vi "Set CUR wrapper.vi"(7 "bAckEna":i32, 8 "error in (no error)":errorcluster caption="错误输入（无错误）", 9 "fCUR":dbl, 10 "dwCanNodeId":u32, 11 "dwDevIndex":u32) -> (0 "error out":errorcluster caption="错误输出", 3 "function return":u32, 4 "pACKInfo out":T1)   [LabVIEW 2016, in "UISimCanFunc_wrapper.lvlib"]
doc: "_declspec (dllexport) DWORD SetCUR_wrapper(DWORD dwDevIndex, DWORD dwCanNodeId, INT iCUR, BOOL bAckEna, P_BASIC_ACK_OBJ pACKInfo);"
uses:
  <userlib>/UISimCanFunc_wrapper/UISimCanFunc_wrapper.lvlib
  <userlib>/UISimCanFunc_wrapper/UISimCanFunc_wrapper.dll
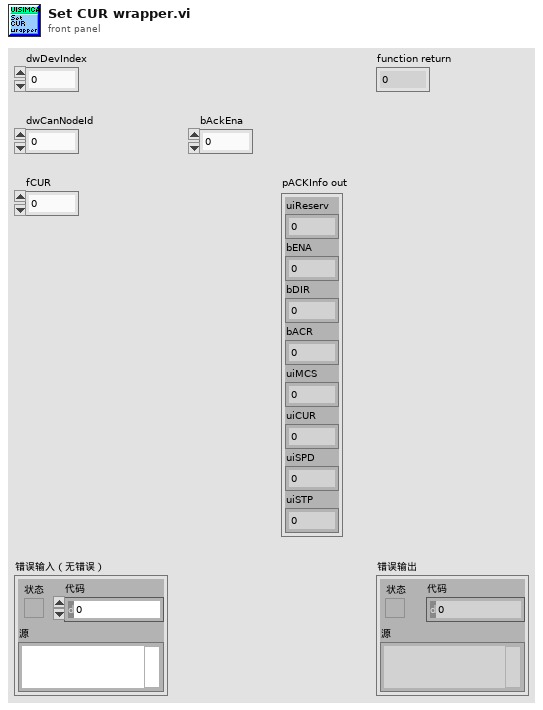
[diagram p1: front panel]
types:
  T1 = cluster{"uiReserv":u32, "bENA":i32, "bDIR":i32, "bACR":i32, "uiMCS":u32, "uiCUR":u32, "uiSPD":u32, "uiSTP":u32}
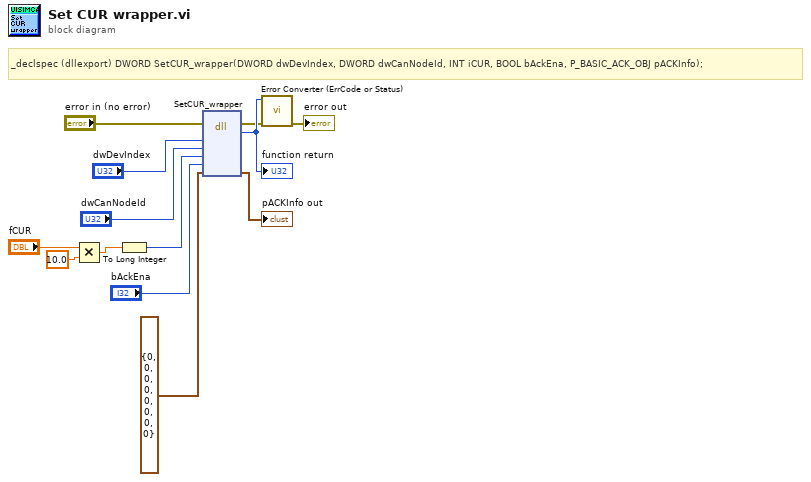
[diagram p0: block diagram]
diagram:
  # "_declspec (dllexport) DWORD SetCUR_wrapper(DWORD dwDevIndex, DWORD dwCanNodeId, INT iCUR, BOOL bAckEna, P_BASIC_ACK_OBJ pACKInfo);"
  n1 = Multiply(x="fCUR", y=10.0) -> (x*y=w2:dbl)
  n2 = To Long Integer(number=w2) -> (32bit integer=w1:i32)
  n3 = dll-call lib="C:/Program Files (x86)/National Instruments/LabVIEW 2016/user.lib/UISimCanFunc_wrapper/UISimCanFunc_wrapper.*" fn="SetCUR_wrapper"(error in="error in (no error)", "dwDevIndex"="dwDevIndex", "dwCanNodeId"="dwCanNodeId", "iCUR"=w1, "bAckEna"="bAckEna", "pACKInfo"=T1 {"uiReserv"=0, "bENA"=0, "bDIR"=0, "bACR"=0, "uiMCS"=0, "uiCUR"=0, "uiSPD"=0, "uiSTP"=0}) -> (error out=w6:errorcluster, w13:u32, "pACKInfo"=→"pACKInfo out":T1)  [unwired: 6 in, 1 out]
  "function return" <- w13
  n4 = call <userlib>:"Error Converter (ErrCode or Status).vi"("error in (no error)"=w6, "error code"=w13) -> ("error out"=→"error out":errorcluster)  [unwired: 9 in]
